vi "Close Connection+.vi"(4 "error in":errorcluster, 7 "Connection":refnum<k7>) -> (0 "error out":errorcluster)   [LabVIEW 2014, in "hse-db.lvlib" / "ADO-DB-Driver.lvlib"]
uses:
  ADO-DB-Driver.lvlib
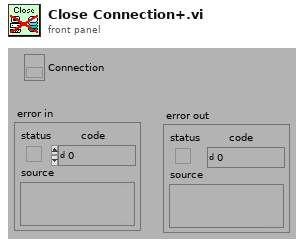
[diagram p1: front panel]
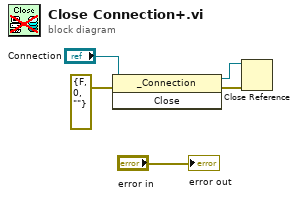
[diagram p0: block diagram]
diagram:
  n1 = invoke class="_Connection" method="Close"(reference="Connection", error in=errorcluster {"status"=FALSE, "code"=0, "source"=""}) -> (reference out=w3:refnum<k7>, error out=w2:errorcluster)  [unwired: 1 in, 1 out]
  n2 = Close Reference(reference=w3, error in (no error)=w2) -> ()  [unwired: 1 out]
  "error out" <- "error in"
